vi "Viavi - typeCast.vi"(6 "Ref Count In":i32, 8 "error in":errorcluster, 9 "Label Name":string, 10 "Input Refnum":refnum<vi>, 11 "Viavi - strictRefs In":T1) -> (0 "error out":errorcluster, 2 "Cast Refnum":refnum<vi>, 3 "Viavi - strictRefs Out":T1, 4 "Ref Count Out":i32)   [LabVIEW 2017]
uses:
  Controls/Viavi - objectRefs.ctl
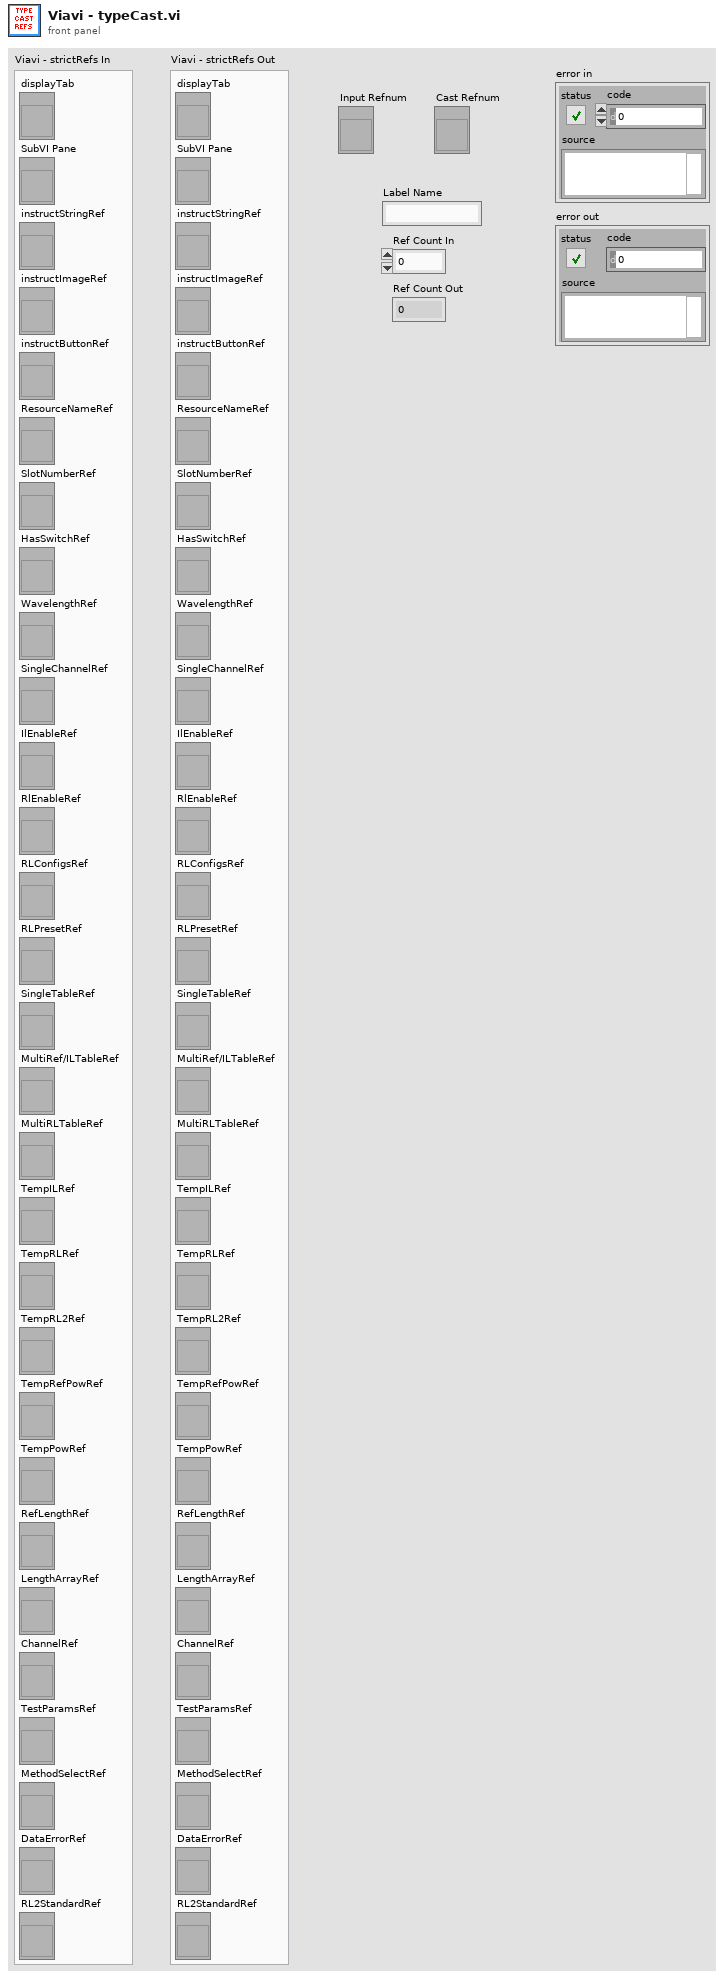
[diagram p1: front panel]
types:
  T1 = typedef "Viavi - objectRefs.ctl" = cluster{"displayTab":refnum<vi>, "SubVI Pane":refnum<vi>, "instructStringRef":refnum<vi>, "instructImageRef":refnum<vi>, "instructButtonRef":refnum<vi>, "ResourceNameRef":refnum<vi>, "SlotNumberRef":refnum<vi>, "HasSwitchRef":refnum<vi>, "WavelengthRef":refnum<vi>, "SingleChannelRef":refnum<vi>, "IlEnableRef":refnum<vi>, "RlEnableRef":refnum<vi>, "RLConfigsRef":refnum<vi>, "RLPresetRef":refnum<vi>, "SingleTableRef":refnum<vi>, "MultiRef/ILTableRef":refnum<vi>, "MultiRLTableRef":refnum<vi>, "TempILRef":refnum<vi>, "TempRLRef":refnum<vi>, "TempRL2Ref":refnum<vi>, "TempRefPowRef":refnum<vi>, "TempPowRef":refnum<vi>, "RefLengthRef":refnum<vi>, "LengthArrayRef":refnum<vi>, "ChannelRef":refnum<vi>, "TestParamsRef":refnum<vi>, "MethodSelectRef":refnum<vi>, "DataErrorRef":refnum<vi>, "RL2StandardRef":refnum<vi>}
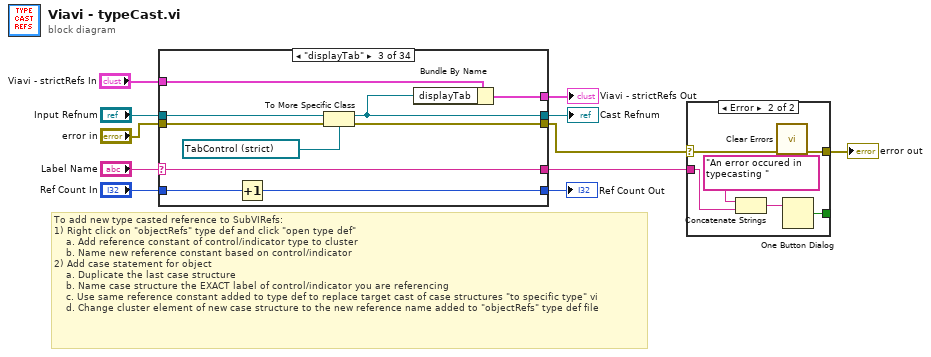
[diagram p0: block diagram]
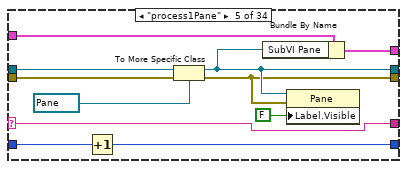
[diagram p6: hidden frame]
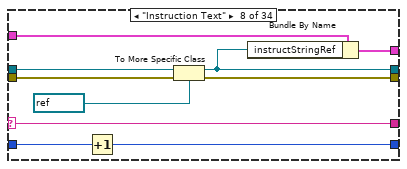
[diagram p9: hidden frame]
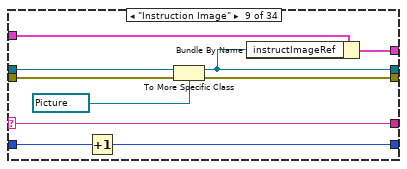
[diagram p10: hidden frame]
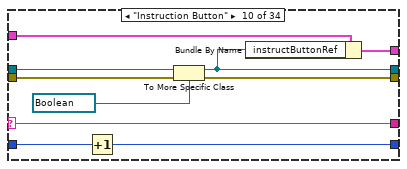
[diagram p11: hidden frame]
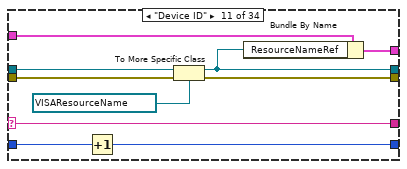
[diagram p12: hidden frame]
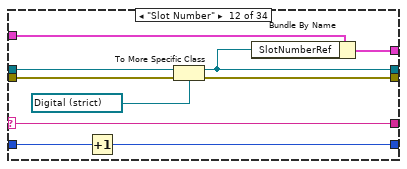
[diagram p13: hidden frame]
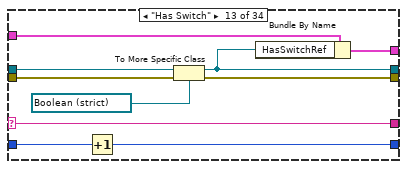
[diagram p14: hidden frame]
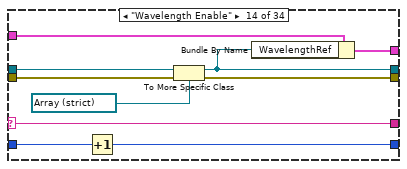
[diagram p15: hidden frame]
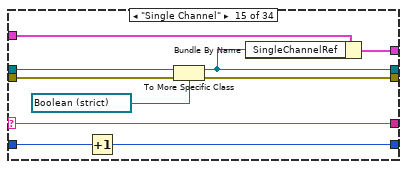
[diagram p16: hidden frame]
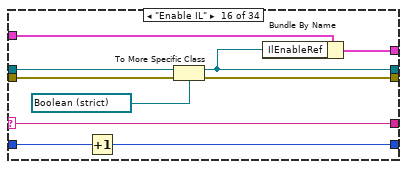
[diagram p17: hidden frame]
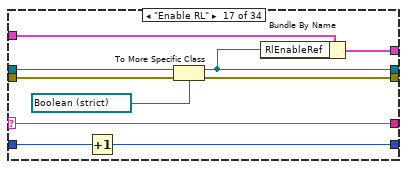
[diagram p18: hidden frame]
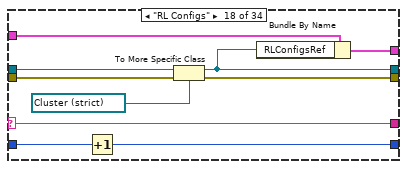
[diagram p19: hidden frame]
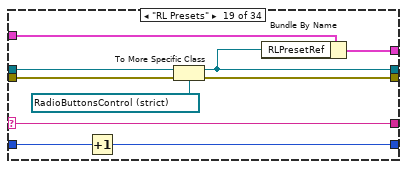
[diagram p20: hidden frame]
diagram:
  # "To add new type casted reference to SubVIRefs:\n1) Right click on \"objectRefs\" type def and click \"open type def\"\n    a. Add reference constant of control/indicator type to cluster\n    b. Name new reference constant based on control/indicator\n2) Add case statement for object\n    a. Duplicate the last case structure\n    b. Name case structure the EXACT label of control/indicator you are referencing\n    c. Use same reference constant added to type def to replace target cast of case structures \"to specific type\" vi\n    d. Change cluster element of new case structure to the new reference name added to \"objectRefs\" type def file"
  n1 = case shown="\"displayTab\"" "Label Name" {
    selector: "Label Name" -> [w12 w17 w23 w32 w37 w48 w53 w58 w68 w79 w88 w98 w108 w118 w128 w138 w148 w159 w169 w178 w188 w198 w208 w218 w228 w238 w248 w258 w268 w278 w289 w299 w309 w319]
    tunnel: "Viavi - strictRefs In" -> [w16 w21 w31 w36 w47 w52 w57 w67 w77 w87 w97 w107 w117 w127 w137 w147 w157 w167 w177 w187 w197 w207 w217 w227 w237 w247 w257 w267 w277 w287 w297 w307 w317 w327]
    tunnel: "Input Refnum" -> [w13 w18 w30 w33 w46 w49 w54 w66 w76 w86 w96 w106 w116 w126 w136 w146 w156 w166 w176 w186 w196 w206 w216 w226 w236 w246 w256 w266 w276 w286 w296 w306 w316 w326]
    tunnel: [w16 w21 w29 w36 w45 w52 w57 w65 w75 w85 w95 w105 w115 w125 w135 w145 w155 w165 w175 w185 w195 w205 w215 w225 w235 w245 w255 w265 w275 w285 w295 w305 w315 w325] -> w7
    tunnel: "error in" -> [w15 w20 w28 w35 w44 w51 w56 w64 w74 w84 w94 w104 w114 w124 w134 w144 w154 w164 w174 w184 w194 w204 w214 w224 w234 w244 w254 w264 w274 w284 w294 w304 w314 w324]
    tunnel: [w15 w20 w24 w35 w38 w51 w56 w60 w70 w80 w90 w100 w110 w120 w130 w140 w150 w160 w170 w180 w190 w200 w210 w220 w230 w240 w250 w260 w270 w280 w290 w300 w310 w320] -> w3
    tunnel: "Ref Count In" -> [w14 w19 w27 w34 w43 w50 w55 w63 w73 w83 w93 w103 w113 w123 w133 w143 w153 w163 w173 w183 w193 w203 w213 w223 w233 w243 w253 w263 w273 w283 w293 w303 w313 w323]
    tunnel: [w14 w19 w26 w34 w42 w50 w55 w62 w72 w82 w92 w102 w112 w122 w132 w142 w152 w162 w172 w182 w192 w202 w212 w222 w232 w242 w252 w262 w272 w282 w292 w302 w312 w322] -> w9
    tunnel: [w13 w18 w25 w33 w39 w49 w54 w61 w71 w81 w91 w101 w111 w121 w131 w141 w151 w161 w171 w181 w191 w201 w211 w221 w231 w241 w251 w261 w271 w281 w291 w301 w311 w321] -> w6
    tunnel: [w12 w17 w23 w32 w37 w48 w53 w58 w68 w79 w88 w98 w108 w118 w128 w138 w148 w159 w169 w178 w188 w198 w208 w218 w228 w238 w248 w258 w268 w278 w289 w299 w309 w319] -> w1
    frame Default {
    }
    frame "-------Tabs-------" {
    }
    frame "displayTab" {
      n2 = Increment(x=w27) -> (x+1=w26:i32)
      n3 = To More Specific Class(target class=refnum<vi> refnum ("displayTab"), reference=w30, error in=w28) -> (specific class reference=w25:refnum<vi>, error out=w24:errorcluster)
      n4 = Bundle By Name(cluster=w31, "displayTab"=w25) -> (w29:T1)
    }
    frame "------Panes------" {
    }
    frame "process1Pane" {
      n5 = Increment(x=w43) -> (x+1=w42:i32)
      n6 = To More Specific Class(target class=refnum<vi> refnum ("displayTab"), reference=w46, error in=w44) -> (specific class reference=w39:refnum<vi>, error out=w38:errorcluster)
      n7 = Bundle By Name(cluster=w47, "SubVI Pane"=w39) -> (w45:T1)
      n8 = property class="Pane"(reference=w39, error in=w38, "Label.Visible"=FALSE) -> ()  [unwired: 2 out]
    }
    frame "-----Splitters-----" {
    }
    frame "-----Objects-----" {
    }
    frame "Instruction Text" {
      n9 = Increment(x=w63) -> (x+1=w62:i32)
      n10 = To More Specific Class(target class=refnum<vi> refnum ("String"), reference=w66, error in=w64) -> (specific class reference=w61:refnum<vi>, error out=w60:errorcluster)
      n11 = Bundle By Name(cluster=w67, "instructStringRef"=w61) -> (w65:T1)
    }
    frame "Instruction Image" {
      n12 = Increment(x=w73) -> (x+1=w72:i32)
      n13 = To More Specific Class(target class=refnum<vi> refnum ("empty picture"), reference=w76, error in=w74) -> (specific class reference=w71:refnum<vi>, error out=w70:errorcluster)
      n14 = Bundle By Name(cluster=w77, "instructImageRef"=w71) -> (w75:T1)
    }
    frame "Instruction Button" {
      n15 = Increment(x=w83) -> (x+1=w82:i32)
      n16 = To More Specific Class(target class=refnum<vi> refnum ("Instruction Button"), reference=w86, error in=w84) -> (specific class reference=w81:refnum<vi>, error out=w80:errorcluster)
      n17 = Bundle By Name(cluster=w87, "instructButtonRef"=w81) -> (w85:T1)
    }
    frame "Device ID" {
      n18 = Increment(x=w93) -> (x+1=w92:i32)
      n19 = To More Specific Class(target class=refnum<vi> refnum ("VISA resource name"), reference=w96, error in=w94) -> (specific class reference=w91:refnum<vi>, error out=w90:errorcluster)
      n20 = Bundle By Name(cluster=w97, "ResourceNameRef"=w91) -> (w95:T1)
    }
    frame "Slot Number" {
      n21 = Increment(x=w103) -> (x+1=w102:i32)
      n22 = To More Specific Class(target class=refnum<vi> refnum ("Ref Count Out"), reference=w106, error in=w104) -> (specific class reference=w101:refnum<vi>, error out=w100:errorcluster)
      n23 = Bundle By Name(cluster=w107, "SlotNumberRef"=w101) -> (w105:T1)
    }
    frame "Has Switch" {
      n24 = Increment(x=w113) -> (x+1=w112:i32)
      n25 = To More Specific Class(target class=refnum<vi> refnum ("Boolean"), reference=w116, error in=w114) -> (specific class reference=w111:refnum<vi>, error out=w110:errorcluster)
      n26 = Bundle By Name(cluster=w117, "HasSwitchRef"=w111) -> (w115:T1)
    }
    frame "Wavelength Enable" {
      n27 = Increment(x=w123) -> (x+1=w122:i32)
      n28 = To More Specific Class(target class=refnum<vi> refnum ("Wavelength Enable"), reference=w126, error in=w124) -> (specific class reference=w121:refnum<vi>, error out=w120:errorcluster)
      n29 = Bundle By Name(cluster=w127, "WavelengthRef"=w121) -> (w125:T1)
    }
    frame "Single Channel" {
      n30 = Increment(x=w133) -> (x+1=w132:i32)
      n31 = To More Specific Class(target class=refnum<vi> refnum ("Boolean"), reference=w136, error in=w134) -> (specific class reference=w131:refnum<vi>, error out=w130:errorcluster)
      n32 = Bundle By Name(cluster=w137, "SingleChannelRef"=w131) -> (w135:T1)
    }
    frame "Enable IL" {
      n33 = Increment(x=w143) -> (x+1=w142:i32)
      n34 = To More Specific Class(target class=refnum<vi> refnum ("Boolean"), reference=w146, error in=w144) -> (specific class reference=w141:refnum<vi>, error out=w140:errorcluster)
      n35 = Bundle By Name(cluster=w147, "IlEnableRef"=w141) -> (w145:T1)
    }
    frame "Enable RL" {
      n36 = Increment(x=w153) -> (x+1=w152:i32)
      n37 = To More Specific Class(target class=refnum<vi> refnum ("Boolean"), reference=w156, error in=w154) -> (specific class reference=w151:refnum<vi>, error out=w150:errorcluster)
      n38 = Bundle By Name(cluster=w157, "RlEnableRef"=w151) -> (w155:T1)
    }
    frame "RL Configs" {
      n39 = Increment(x=w163) -> (x+1=w162:i32)
      n40 = To More Specific Class(target class=refnum<vi> refnum ("RL Configs"), reference=w166, error in=w164) -> (specific class reference=w161:refnum<vi>, error out=w160:errorcluster)
      n41 = Bundle By Name(cluster=w167, "RLConfigsRef"=w161) -> (w165:T1)
    }
    frame "RL Presets" {
      n42 = Increment(x=w173) -> (x+1=w172:i32)
      n43 = To More Specific Class(target class=refnum<vi> refnum ("RL Presets"), reference=w176, error in=w174) -> (specific class reference=w171:refnum<vi>, error out=w170:errorcluster)
      n44 = Bundle By Name(cluster=w177, "RLPresetRef"=w171) -> (w175:T1)
    }
    frame "Single Table" {
      n45 = Increment(x=w183) -> (x+1=w182:i32)
      n46 = To More Specific Class(target class=refnum<vi> refnum ("Single Table"), reference=w186, error in=w184) -> (specific class reference=w181:refnum<vi>, error out=w180:errorcluster)
      n47 = Bundle By Name(cluster=w187, "SingleTableRef"=w181) -> (w185:T1)
    }
    frame "Multi Ref/IL Table" {
      n48 = Increment(x=w193) -> (x+1=w192:i32)
      n49 = To More Specific Class(target class=refnum<vi> refnum ("Single Table"), reference=w196, error in=w194) -> (specific class reference=w191:refnum<vi>, error out=w190:errorcluster)
      n50 = Bundle By Name(cluster=w197, "MultiRef/ILTableRef"=w191) -> (w195:T1)
    }
    frame "Multi RL Table" {
      n51 = Increment(x=w203) -> (x+1=w202:i32)
      n52 = To More Specific Class(target class=refnum<vi> refnum ("Single Table"), reference=w206, error in=w204) -> (specific class reference=w201:refnum<vi>, error out=w200:errorcluster)
      n53 = Bundle By Name(cluster=w207, "MultiRLTableRef"=w201) -> (w205:T1)
    }
    frame "Channel Select" {
      n54 = Increment(x=w213) -> (x+1=w212:i32)
      n55 = To More Specific Class(target class=refnum<vi> refnum ("Wavelength Enable"), reference=w216, error in=w214) -> (specific class reference=w211:refnum<vi>, error out=w210:errorcluster)
      n56 = Bundle By Name(cluster=w217, "ChannelRef"=w211) -> (w215:T1)
    }
    frame "Temp IL Array" {
      n57 = Increment(x=w223) -> (x+1=w222:i32)
      n58 = To More Specific Class(target class=refnum<vi> refnum ("Temp IL Array"), reference=w226, error in=w224) -> (specific class reference=w221:refnum<vi>, error out=w220:errorcluster)
      n59 = Bundle By Name(cluster=w227, "TempILRef"=w221) -> (w225:T1)
    }
    frame "Temp RL Array" {
      n60 = Increment(x=w233) -> (x+1=w232:i32)
      n61 = To More Specific Class(target class=refnum<vi> refnum ("Temp IL Array"), reference=w236, error in=w234) -> (specific class reference=w231:refnum<vi>, error out=w230:errorcluster)
      n62 = Bundle By Name(cluster=w237, "TempRLRef"=w231) -> (w235:T1)
    }
    frame "Temp RL2 Array" {
      n63 = Increment(x=w243) -> (x+1=w242:i32)
      n64 = To More Specific Class(target class=refnum<vi> refnum ("Temp IL Array"), reference=w246, error in=w244) -> (specific class reference=w241:refnum<vi>, error out=w240:errorcluster)
      n65 = Bundle By Name(cluster=w247, "TempRL2Ref"=w241) -> (w245:T1)
    }
    frame "Temp Ref Power Array" {
      n66 = Increment(x=w253) -> (x+1=w252:i32)
      n67 = To More Specific Class(target class=refnum<vi> refnum ("Temp IL Array"), reference=w256, error in=w254) -> (specific class reference=w251:refnum<vi>, error out=w250:errorcluster)
      n68 = Bundle By Name(cluster=w257, "TempRefPowRef"=w251) -> (w255:T1)
    }
    frame "Temp Power Array" {
      n69 = Increment(x=w263) -> (x+1=w262:i32)
      n70 = To More Specific Class(target class=refnum<vi> refnum ("Temp IL Array"), reference=w266, error in=w264) -> (specific class reference=w261:refnum<vi>, error out=w260:errorcluster)
      n71 = Bundle By Name(cluster=w267, "TempPowRef"=w261) -> (w265:T1)
    }
    frame "Ref Length Array" {
      n72 = Increment(x=w273) -> (x+1=w272:i32)
      n73 = To More Specific Class(target class=refnum<vi> refnum ("Temp IL Array"), reference=w276, error in=w274) -> (specific class reference=w271:refnum<vi>, error out=w270:errorcluster)
      n74 = Bundle By Name(cluster=w277, "RefLengthRef"=w271) -> (w275:T1)
    }
    frame "Length Array" {
      n75 = Increment(x=w283) -> (x+1=w282:i32)
      n76 = To More Specific Class(target class=refnum<vi> refnum ("Temp IL Array"), reference=w286, error in=w284) -> (specific class reference=w281:refnum<vi>, error out=w280:errorcluster)
      n77 = Bundle By Name(cluster=w287, "LengthArrayRef"=w281) -> (w285:T1)
    }
    frame "Testing Parameters" {
      n78 = Increment(x=w293) -> (x+1=w292:i32)
      n79 = To More Specific Class(target class=refnum<vi> refnum ("TestParamsRef"), reference=w296, error in=w294) -> (specific class reference=w291:refnum<vi>, error out=w290:errorcluster)
      n80 = Bundle By Name(cluster=w297, "TestParamsRef"=w291) -> (w295:T1)
    }
    frame "Method Selection" {
      n81 = Increment(x=w303) -> (x+1=w302:i32)
      n82 = To More Specific Class(target class=refnum<vi> refnum ("Method Selection"), reference=w306, error in=w304) -> (specific class reference=w301:refnum<vi>, error out=w300:errorcluster)
      n83 = Bundle By Name(cluster=w307, "MethodSelectRef"=w301) -> (w305:T1)
    }
    frame "Data Error" {
      n84 = Increment(x=w313) -> (x+1=w312:i32)
      n85 = To More Specific Class(target class=refnum<vi> refnum ("Data Error"), reference=w316, error in=w314) -> (specific class reference=w311:refnum<vi>, error out=w310:errorcluster)
      n86 = Bundle By Name(cluster=w317, "DataErrorRef"=w311) -> (w315:T1)
    }
    frame "RL2 Standard" {
      n87 = Increment(x=w323) -> (x+1=w322:i32)
      n88 = To More Specific Class(target class=refnum<vi> refnum ("RL2 Standard"), reference=w326, error in=w324) -> (specific class reference=w321:refnum<vi>, error out=w320:errorcluster)
      n89 = Bundle By Name(cluster=w327, "RL2StandardRef"=w321) -> (w325:T1)
    }
  }
  "Ref Count Out" <- w9
  "Viavi - strictRefs Out" <- w7
  "Cast Refnum" <- w6
  n90 = case shown="Error" w3 {
    selector: w3 -> [w328 w334]
    tunnel: [w328 w333] -> w2
    tunnel: w1 -> [_ w331]
    tunnel: [_ w329] -> _
    frame No Error {
    }
    frame Error {
      n91 = Concatenate Strings("An error occured in typecasting ", w331) -> (w330:string)
      n92 = call <vilib>:"Clear Errors.vi"("error in (no error)"=w334) -> ("error out"=w333:errorcluster)  [unwired: 5 in, 1 out]
      n93 = One Button Dialog(message=w330) -> (true=w329:bool)  [unwired: 1 in]
    }
  }
  "error out" <- w2
